vi "轮速控制（新）.vi"(2 "速度":dbl[](array[numeric])=[0.0, 0.0, 0.0, 0.0]) -> (0 "错误输出":errorcluster)   [LabVIEW 2016]
uses:
  <vilib>/myRIO/Instrument Drivers/Onboard IO/PWM/PWM.lvlib
  <vilib>/myRIO/Instrument Drivers/Onboard IO/DIO/DIO.lvlib
panel:
  in  "停止":bool
  in  "error in  2":errorcluster
  out "添加的数组 2":bool[](array[boolean])
  out "添加的数组":bool[](array[boolean])
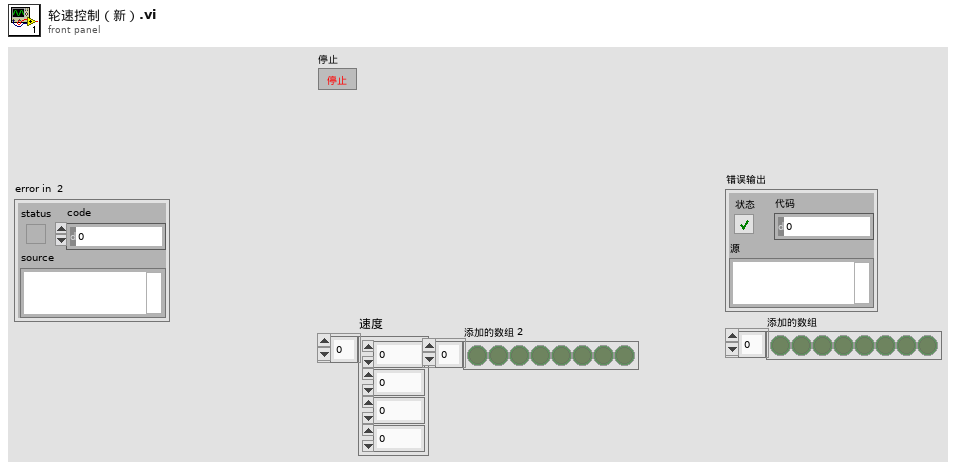
[diagram p1: front panel]
types:
  T1 = typedef "PWM.lvlib/PWM Reference.ctl" = cluster{"myRIO Reference":T2, "PWM Channels Enum":T6, "PWM Configuration":T7}
  T2 = typedef "myRIO Generic Hardware Reference.ctl" = cluster{"myRIO Model":T3, "myRIO Hardware Reference":T4}
  T3 = typedef "Hardware Version Enum.ctl" = enum16{"Unknown", "myRIO-1900", "myRIO-1950", "roboRIO", "NI ELVIS RIO CM"}
  T4 = typedef "myRIO v1.0 Reference.ctl" = cluster{"Generic FPGA Reference":T5, "Allow multiple opens":bool}
  T5 = typedef "Generic FPGA Reference.ctl" = refnum<k20>
  T6 = typedef "PWM Channels Enum.ctl" = enum16{"Not Connected", "C/PWM0", "C/PWM1", "A/PWM0", "A/PWM1", "A/PWM2", "B/PWM0", "B/PWM1", "B/PWM2", "PWM/PWM0", "PWM/PWM1", "PWM/PWM2", "PWM/PWM3", "PWM/PWM4", "PWM/PWM5", "PWM/PWM6", "PWM/PWM7", "PWM/PWM8", "PWM/PWM9"}
  T7 = typedef "PWM.lvlib/PWM Configuration.ctl" = cluster{"Frequency":dbl, "Duty Cycle":dbl}
  T8 = typedef "DIO.lvlib/DIO Reference.ctl" = cluster{"myRIO Reference":T2, "DIO Channels List":T9}
  T9 = typedef "DIO Channels List.ctl" = T10[]
  T10 = typedef "DIO Channels Enum.ctl" = enum16{"Not Connected", "C/DIO0", "C/DIO1", "C/DIO2", "C/DIO3", "C/DIO4", "C/DIO5", "C/DIO6", "C/DIO7", "A/DIO0", "A/DIO1", "A/DIO2", "A/DIO3", "A/DIO4", "A/DIO5", "A/DIO6", "A/DIO7", "A/DIO8", "A/DIO9", "A/DIO10", "A/DIO11", "A/DIO12", "A/DIO13", "A/DIO14", "A/DIO15", "B/DIO0", "B/DIO1", "B/DIO2", "B/DIO3", "B/DIO4", "B/DIO5", "B/DIO6", "B/DIO7", "B/DIO8", "B/DIO9", "B/DIO10", "B/DIO11", "B/DIO12", "B/DIO13", "B/DIO14", "B/DIO15", "LED0", "LED1", "LED2", "LED3", "Button0", "DIO/DIO0", "DIO/DIO1", "DIO/DIO2", "DIO/DIO3", "DIO/DIO4", "DIO/DIO5", "DIO/DIO6", "DIO/DIO7", "DIO/DIO8", "DIO/DIO9", "SPI/CS0", "SPI/CS1", "SPI/CS2", "SPI/CS3", "LED RADIO (Green)", "LED RADIO (Red)", "LED COMM (Green)", "LED COMM (Red)", "LED MODE (Green)", "LED MODE (Red)"}
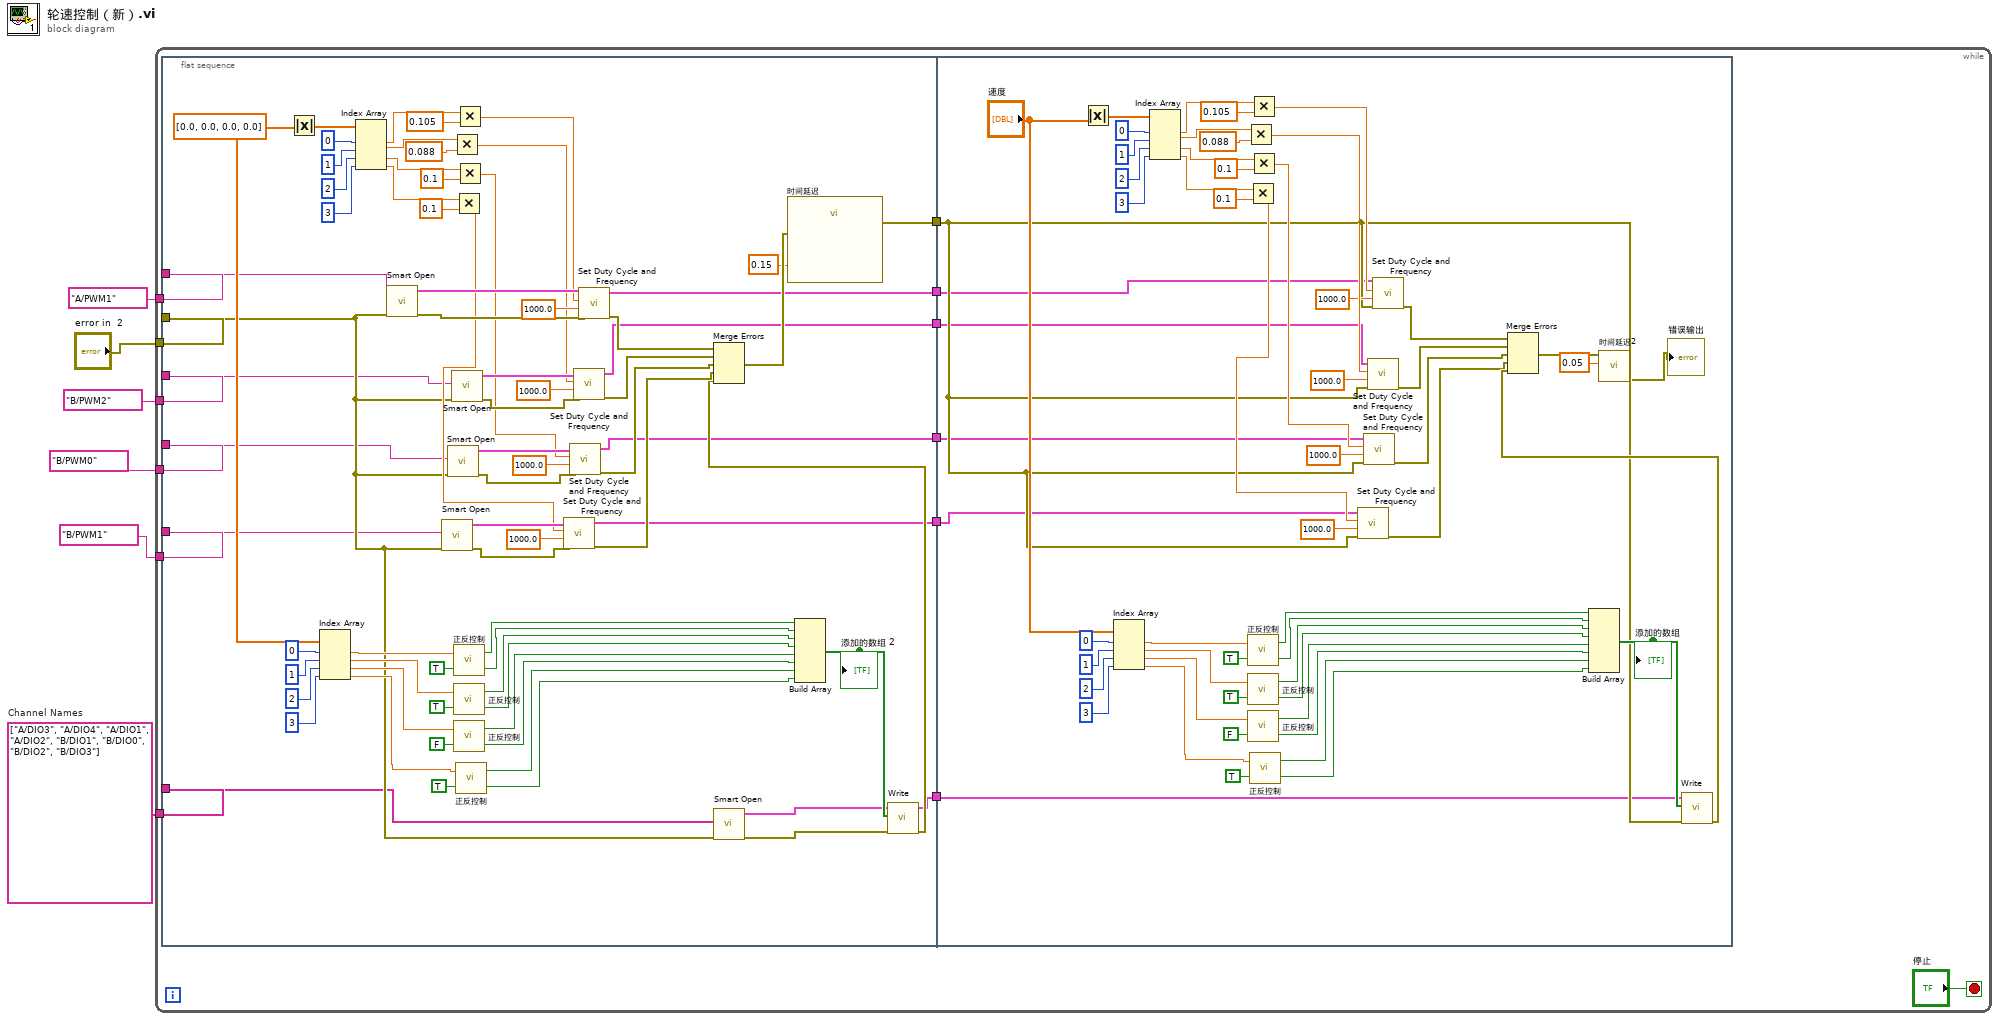
[diagram p0: block diagram]
diagram:
  w1 = tag[] ["A/DIO3", "A/DIO4", "A/DIO1", "A/DIO2", "B/DIO1", "B/DIO0", "B/DIO2", "B/DIO3"]  # Channel Names
  n1 = while {
    tunnel: tag "A/PWM1" ("Channel Name") -> [w12]
    tunnel: tag "B/PWM2" ("Channel Name") -> [w11]
    tunnel: tag "B/PWM0" ("Channel Name") -> [w10]
    tunnel: tag "B/PWM1" ("Channel Name") -> [w9]
    tunnel: "error in  2" -> [w8]
    tunnel: w1 -> [w7]
    stop <- "停止" stop-if-true
    n2 = flat-sequence {
      tunnel: [w32] -> w19
      tunnel: [w30] -> w18
      tunnel: [w29] -> w17
      tunnel: [w28] -> w16
      tunnel: [w27] -> w15
      tunnel: w8 -> [w26]
      tunnel: [w25] -> w14
      tunnel: w12 -> [w24]
      tunnel: w11 -> [w23]
      tunnel: w10 -> [w22]
      tunnel: w9 -> [w21]
      tunnel: w7 -> [w20]
      tunnel: w19 -> [w100]
      tunnel: w18 -> [w99]
      tunnel: w17 -> [w98]
      tunnel: w16 -> [w97]
      tunnel: w15 -> [w96]
      tunnel: w14 -> [w95]
      frame #0 {
        w54 = dbl[] [0.0, 0.0, 0.0, 0.0] ("速度 2")
        n3 = Absolute Value(x=w54) -> (abs(x)=w63:dbl[])
        n4 = Index Array(array=w54, index #1=0 ("索引"), index #2=1 ("索引"), index #3=2 ("索引"), index #4=3 ("索引")) -> (element #1=w53:dbl, element #2=w48:dbl, element #3=w47:dbl, element #4=w46:dbl)
        n5 = Index Array(array=w63, index #1=0 ("索引"), index #2=1 ("索引"), index #3=2 ("索引"), index #4=3 ("索引")) -> (element #1=w71:dbl, element #2=w70:dbl, element #3=w69:dbl, element #4=w68:dbl)
        n6 = call <vilib>:"Smart Open.vi"("error in (no error)"=w26, "Channel Name"=w24) -> ("error out"=w83:errorcluster, "PWM Ref Out"=w91:T1)  [unwired: 8 in]
        n7 = call <vilib>:"Smart Open.vi"("error in (no error)"=w26, "Channel Name"=w21) -> ("error out"=w80:errorcluster, "PWM Ref Out"=w85:T1)  [unwired: 8 in]
        n8 = call <vilib>:"Smart Open.vi"("error in (no error)"=w26, "Channel Name"=w22) -> ("error out"=w81:errorcluster, "PWM Ref Out"=w87:T1)  [unwired: 8 in]
        n9 = Multiply(x=w70, y=0.088) -> (x*y=w61:dbl)
        n10 = call <vilib>:"Smart Open.vi"("error in (no error)"=w26, "Channel Name"=w23) -> ("error out"=w82:errorcluster, "PWM Ref Out"=w89:T1)  [unwired: 8 in]
        n11 = Multiply(x=w68, y=0.1) -> (x*y=w59:dbl)
        n12 = call "正反控制.vi"("接法"=TRUE, "x"=w53) -> ("INB"=w41:bool, "INA"=w42:bool)
        n13 = call "正反控制.vi"("接法"=TRUE, "x"=w48) -> ("INB"=w39:bool, "INA"=w40:bool)
        n14 = call "正反控制.vi"("接法"=FALSE, "x"=w47) -> ("INB"=w37:bool, "INA"=w38:bool)
        n15 = Multiply(x=w71, y=0.105) -> (x*y=w62:dbl)
        n16 = Multiply(x=w69, y=0.1) -> (x*y=w60:dbl)
        n17 = call "正反控制.vi"("接法"=TRUE, "x"=w46) -> ("INB"=w35:bool, "INA"=w36:bool)
        n18 = call <vilib>:"Set Duty Cycle and Frequency.vi"("error in (no error)"=w80, "Frequency [Hz]"=1000.0, "Duty Cycle"=w59, "PWM Ref In"=w85) -> ("error out"=w76:errorcluster, "PWM Ref Out"=w27:T1)  [unwired: 5 in]
        n19 = call <vilib>:"Set Duty Cycle and Frequency.vi"("error in (no error)"=w81, "Frequency [Hz]"=1000.0, "Duty Cycle"=w60, "PWM Ref In"=w87) -> ("error out"=w77:errorcluster, "PWM Ref Out"=w28:T1)  [unwired: 5 in]
        n20 = call <vilib>:"Set Duty Cycle and Frequency.vi"("error in (no error)"=w82, "Frequency [Hz]"=1000.0, "Duty Cycle"=w61, "PWM Ref In"=w89) -> ("error out"=w78:errorcluster, "PWM Ref Out"=w29:T1)  [unwired: 5 in]
        n21 = call <vilib>:"Set Duty Cycle and Frequency.vi"("error in (no error)"=w83, "Frequency [Hz]"=1000.0, "Duty Cycle"=w62, "PWM Ref In"=w91) -> ("error out"=w79:errorcluster, "PWM Ref Out"=w30:T1)  [unwired: 5 in]
        n22 = call <vilib>:"Smart Open.vi"("error in (no error)"=w26, "Channel Names"=w20) -> ("error out"=w43:errorcluster, "DIO Ref Out"=w44:T8)  [unwired: 8 in]
        n23 = Build Array(w42, w41, w40, w39, w38, w37, w36, w35) -> (w45:bool[])
        "添加的数组 2" <- w45
        n24 = call <vilib>:"Write.vi"("error in (no error)"=w43, "Values"=w45, "DIO Ref In"=w44) -> ("error out"=w34:errorcluster, "DIO Ref Out"=w25:T8)  [unwired: 6 in]
        n25 = Merge Errors(w79, w78, w77, w76, w34) -> (w33:errorcluster)
        n26 = call "时间延迟"("error in (no error)"=w33, "Delay Time (s)"=0.15) -> ("error out"=w32:errorcluster)  [unwired: 9 in]
      }
      frame #1 {
        n27 = Absolute Value(x="速度") -> (abs(x)=w121:dbl[])
        n28 = Index Array(array="速度", index #1=0 ("索引"), index #2=1 ("索引"), index #3=2 ("索引"), index #4=3 ("索引")) -> (element #1=w131:dbl, element #2=w136:dbl, element #3=w137:dbl, element #4=w138:dbl)
        n29 = Index Array(array=w121, index #1=0 ("索引"), index #2=1 ("索引"), index #3=2 ("索引"), index #4=3 ("索引")) -> (element #1=w113:dbl, element #2=w114:dbl, element #3=w115:dbl, element #4=w116:dbl)
        n30 = Multiply(x=w114, y=0.088) -> (x*y=w123:dbl)
        n31 = Multiply(x=w116, y=0.1) -> (x*y=w125:dbl)
        n32 = call "正反控制.vi"("接法"=TRUE, "x"=w131) -> ("INB"=w141:bool, "INA"=w140:bool)
        n33 = call "正反控制.vi"("接法"=TRUE, "x"=w136) -> ("INB"=w143:bool, "INA"=w142:bool)
        n34 = call "正反控制.vi"("接法"=FALSE, "x"=w137) -> ("INB"=w145:bool, "INA"=w144:bool)
        n35 = Multiply(x=w113, y=0.105) -> (x*y=w122:dbl)
        n36 = Multiply(x=w115, y=0.1) -> (x*y=w124:dbl)
        n37 = call "正反控制.vi"("接法"=TRUE, "x"=w138) -> ("INB"=w147:bool, "INA"=w146:bool)
        n38 = call <vilib>:"Set Duty Cycle and Frequency.vi"("error in (no error)"=w100, "Frequency [Hz]"=1000.0, "Duty Cycle"=w125, "PWM Ref In"=w96) -> ("error out"=w108:errorcluster)  [unwired: 5 in, 1 out]
        n39 = call <vilib>:"Set Duty Cycle and Frequency.vi"("error in (no error)"=w100, "Frequency [Hz]"=1000.0, "Duty Cycle"=w124, "PWM Ref In"=w97) -> ("error out"=w107:errorcluster)  [unwired: 5 in, 1 out]
        n40 = call <vilib>:"Set Duty Cycle and Frequency.vi"("error in (no error)"=w100, "Frequency [Hz]"=1000.0, "Duty Cycle"=w123, "PWM Ref In"=w98) -> ("error out"=w106:errorcluster)  [unwired: 5 in, 1 out]
        n41 = call <vilib>:"Set Duty Cycle and Frequency.vi"("error in (no error)"=w100, "Frequency [Hz]"=1000.0, "Duty Cycle"=w122, "PWM Ref In"=w99) -> ("error out"=w105:errorcluster)  [unwired: 5 in, 1 out]
        n42 = Build Array(w140, w141, w142, w143, w144, w145, w146, w147) -> (w139:bool[])
        "添加的数组" <- w139
        n43 = call <vilib>:"Write.vi"("error in (no error)"=w100, "Values"=w139, "DIO Ref In"=w95) -> ("error out"=w148:errorcluster)  [unwired: 6 in, 1 out]
        n44 = Merge Errors(w105, w106, w107, w108, w148) -> (w94:errorcluster)
        n45 = call "时间延迟2"("error in (no error)"=w94, "Delay Time (s)"=0.05) -> ("error out"=→"错误输出":errorcluster)  [unwired: 9 in]
      }
    }
  }
